vi "fromXML.vi"(8 "error in (no error)":errorcluster, 10 "channel_configXML":refnum<class "xmlNode.lvclass">, 11 "RfOutputChannel in":refnum<class "RfOutputChannel.lvclass">) -> (0 "error out":errorcluster, 3 "RfOutputChannel out":refnum<class "RfOutputChannel.lvclass">)   [LabVIEW 2009, in "Tools.lvlib" / "DatabaseHelpers.lvlib" / "RfOutputChannel.lvclass"]
uses:
  RfOutputChannel.lvclass
  xmlNode/xmlNode.lvclass
  RfOutputChannel.lvclass/RfOutputChannel.ctl
  Channel.lvclass
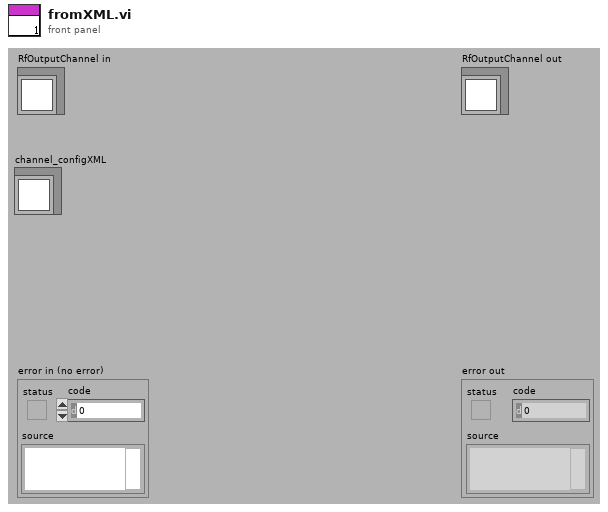
[diagram p1: front panel]
types:
  T1 = cluster{"attribute string":string, "stringValue":string}
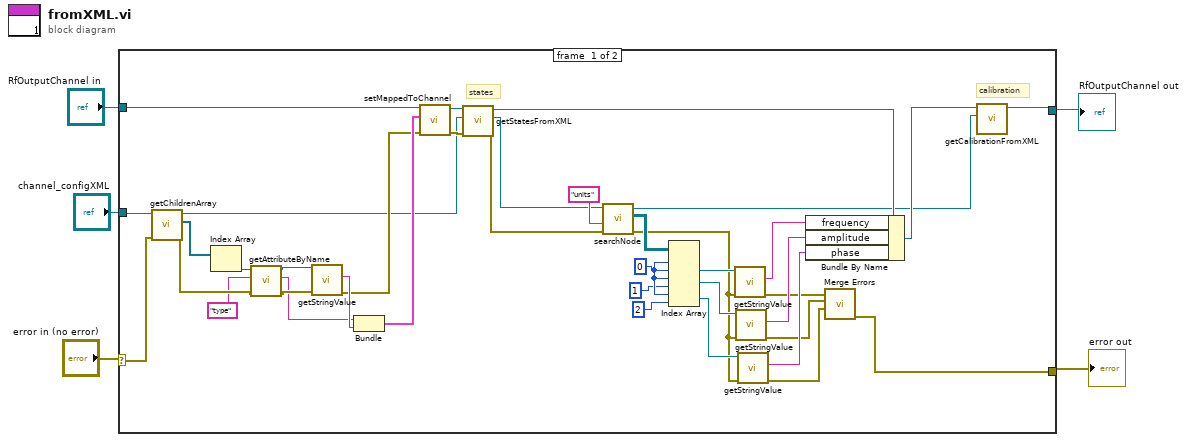
[diagram p0: block diagram]
diagram:
  n1 = case shown="No Error" "error in (no error)" {
    selector: "error in (no error)" -> [w10 w44]
    tunnel: [w23 w44] -> w5
    tunnel: [w22 w45] -> w2
    tunnel: "channel_configXML" -> [w11 _]
    tunnel: "RfOutputChannel in" -> [w8 w45]
    frame #0 {
      w41 = 0
      # "calibration"
      # "states"
      n2 = call-dynamic "getChildrenArray.vi"("error in (no error)"=w10, "xmlNode.lvclass in"=w11) -> ("error out"=w17:errorcluster, "Children"=w18:refnum<class "xmlNode.lvclass">[], "xmlNode.lvclass out"=w6:refnum<class "xmlNode.lvclass">)  [unwired: 7 in]
      n3 = Index Array(array=w18) -> (element=w16:refnum<class "xmlNode.lvclass">)  [unwired: 1 in]
      n4 = call-dynamic "getAttributeByName.vi"("error in (no error)"=w17, "AttributeName"="type", "xmlNode in"=w16) -> ("error out"=w14:errorcluster, "attribute string"=w13:string, "xmlNode out"=w15:refnum<class "xmlNode.lvclass">)  [unwired: 6 in]
      n5 = call-dynamic "getStringValue.vi"("error in (no error)"=w14, "xmlNode.lvclass in"=w15) -> ("error out"=w19:errorcluster, "stringValue"=w21:string)  [unwired: 7 in, 1 out]
      n6 = Bundle("attribute string"=w13, "stringValue"=w21) -> (w20:T1)  [unwired: 1 in]
      n7 = call "setMappedToChannel.vi"("error in (no error)"=w19, "mappedTo"=w20, "Channel.lvclass in"=w8) -> ("error out"=w7:errorcluster, "Channel.lvclass out"=w9:refnum<class "RfOutputChannel.lvclass">)  [unwired: 7 in]
      n8 = call-dynamic "getStatesFromXML.vi"("error in (no error)"=w7, "channel_configXML"=w6, "RfOutputChannel in"=w9) -> ("error out"=w26:errorcluster, "channel_configXML out"=w27:refnum<class "xmlNode.lvclass">, "RfOutputChannel out"=w28:refnum<class "RfOutputChannel.lvclass">)  [unwired: 6 in]
      n9 = call-dynamic "searchNode.vi"("error in (no error)"=w26, "searchElementName"="units", "xmlNode in"=w27) -> ("error out"=w35:errorcluster, "arrayXmlNodes"=w42:refnum<class "xmlNode.lvclass">[][], "xmlNode out"=w24:refnum<class "xmlNode.lvclass">)  [unwired: 6 in]
      n10 = Index Array(array=w42, index (row) #1=w41, index (col) #1=w41, index (row) #2=w41, index (col) #2=1, index (row) #3=w41, index (col) #3=2) -> (element #1=w38:refnum<class "xmlNode.lvclass">, element #2=w37:refnum<class "xmlNode.lvclass">, element #3=w36:refnum<class "xmlNode.lvclass">)
      n11 = call-dynamic "getStringValue.vi"("error in (no error)"=w35, "xmlNode.lvclass in"=w38) -> ("error out"=w31:errorcluster, "stringValue"=w32:string)  [unwired: 7 in, 1 out]
      n12 = call-dynamic "getStringValue.vi"("error in (no error)"=w35, "xmlNode.lvclass in"=w37) -> ("error out"=w30:errorcluster, "stringValue"=w33:string)  [unwired: 7 in, 1 out]
      n13 = call-dynamic "getStringValue.vi"("error in (no error)"=w35, "xmlNode.lvclass in"=w36) -> ("error out"=w29:errorcluster, "stringValue"=w34:string)  [unwired: 7 in, 1 out]
      n14 = Bundle By Name(cluster=w28, "frequency"=w32, "amplitude"=w33, "phase"=w34) -> (w25:refnum<class "RfOutputChannel.lvclass">)
      n15 = call <vilib>:"Merge Errors.vi"("error in 3 (no error)"=w29, "error in 2 (no error)"=w30, "error in 1 (no error)"=w31) -> ("error out"=w23:errorcluster)  [unwired: 4 in]
      n16 = call-dynamic "getCalibrationFromXML.vi"("channel_configXML"=w24, "RfOutputChannel in"=w25) -> ("RfOutputChannel out"=w22:refnum<class "RfOutputChannel.lvclass">)  [unwired: 7 in, 2 out]
    }
    frame #1 {
    }
  }
  "error out" <- w5
  "RfOutputChannel out" <- w2
